vi "Indexed Read.vi"(8 "Index In":i32, 10 "timeout in ms (60 sec)":i32=60000, 11 "Future in":refnum<class "Future.lvclass">) -> (0 "error out":errorcluster, 1 "Result Error":errorcluster, 2 "Result Value":variant, 3 "Index Out":i32, 4 "Timed Out":bool)   [LabVIEW 2017, in "Futures.lvlib" / "Future.lvclass"]
uses:
  Future.lvclass
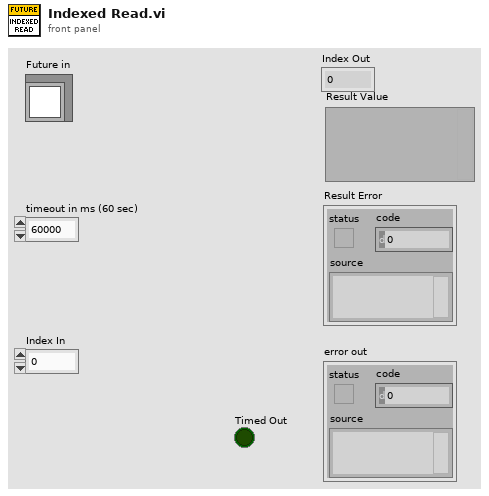
[diagram p1: front panel]
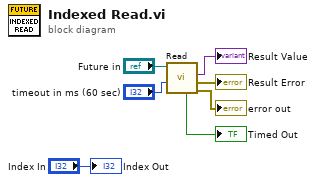
[diagram p0: block diagram]
diagram:
  n1 = call "Read.vi"("timeout in ms (60 sec)"="timeout in ms (60 sec)", "Future in"="Future in") -> ("error out"=→"error out":errorcluster, "Result Error"=→"Result Error":errorcluster, "Result Value"=→"Result Value":variant, "Timed Out"=→"Timed Out":bool)  [unwired: 6 in]
  "Index Out" <- "Index In"
